vi "Coord window-Set motor coordinates colour.vi"(8 "error in (no error)":errorcluster) -> (0 "error out":errorcluster)   [LabVIEW 2013]
uses:
  Globals/Coord window-Globals.vi
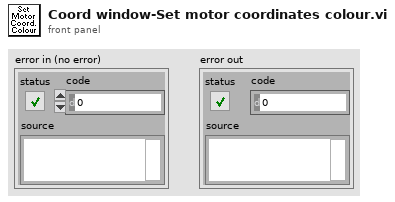
[diagram p1: front panel]
types:
  T1 = typedef "Coordinate list window refs.ctl" = cluster{"Window Name (i.e. Key)":string, "menu reference":refnum<k9>, "VI's reference":refnum<vi>, "Pane 1":refnum<vi>, "Pane 2":refnum<vi>, "Coord Listbox":refnum<vi>, "File name":refnum<vi>, "Picture Map":refnum<vi>, "Stage XYZ Position ind.":refnum<vi>}
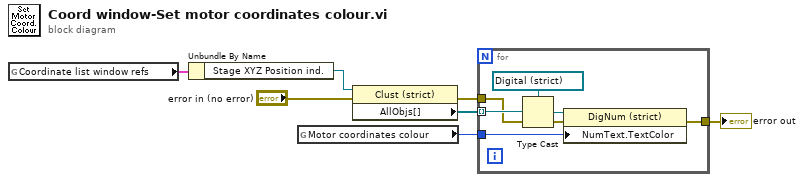
[diagram p0: block diagram]
diagram:
  n1 = global read "Coord window-Globals.vi" "Coordinate list window refs"() -> (w2:T1)
  n2 = Unbundle By Name(w2) -> ("Stage XYZ Position ind."=w1:refnum<vi>)
  n3 = global read "Coord window-Globals.vi" "Motor coordinates colour"() -> (w4:u32)
  n4 = property on="Property Node" class="Clust (strict)"(reference=w1, error in="error in (no error)") -> (error out=w6:errorcluster, "AllObjs[]"=w3:refnum<vi>[])  [unwired: 1 out]
  n5 = for {
    tunnel: w3 -> [w12] mode=indexing
    tunnel: w4 -> [w11]
    tunnel: [w9] -> w5
    tunnel: w6 -> [w8]
    n6 = Type Cast(type=refnum<vi> refnum ("Y"), x=w12) -> (*(type *) &x=w10:refnum<vi>)
    n7 = property class="DigNum (strict)"(reference=w10, error in=w8, "NumText.TextColor"=w11) -> (error out=w9:errorcluster)  [unwired: 1 out]
  }
  "error out" <- w5
